vi "555集成定时器组成单稳态触发器.vi"() -> ()   [LabVIEW 2018]
panel:
  out "V":dbl
  out "毫秒计时值":u32
  out "波形图表":cluster{i16, i16}(graph)
  in  "确定按钮":bool
  in  "C值":dbl
  in  "R值":dbl
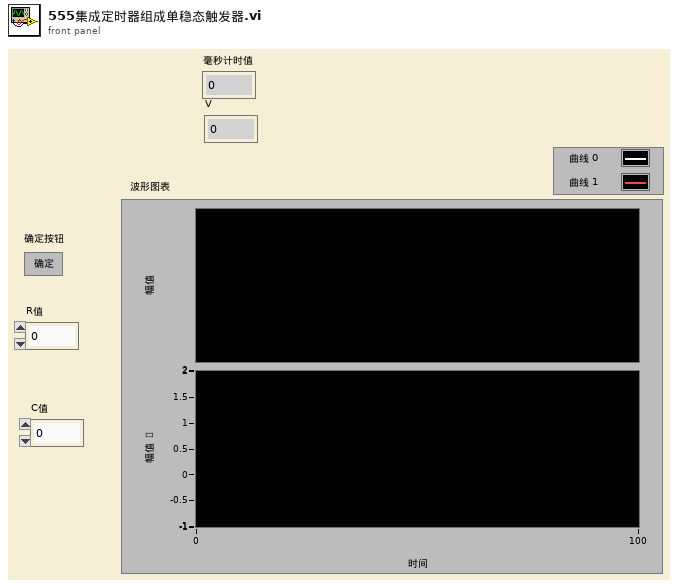
[diagram p1: front panel]
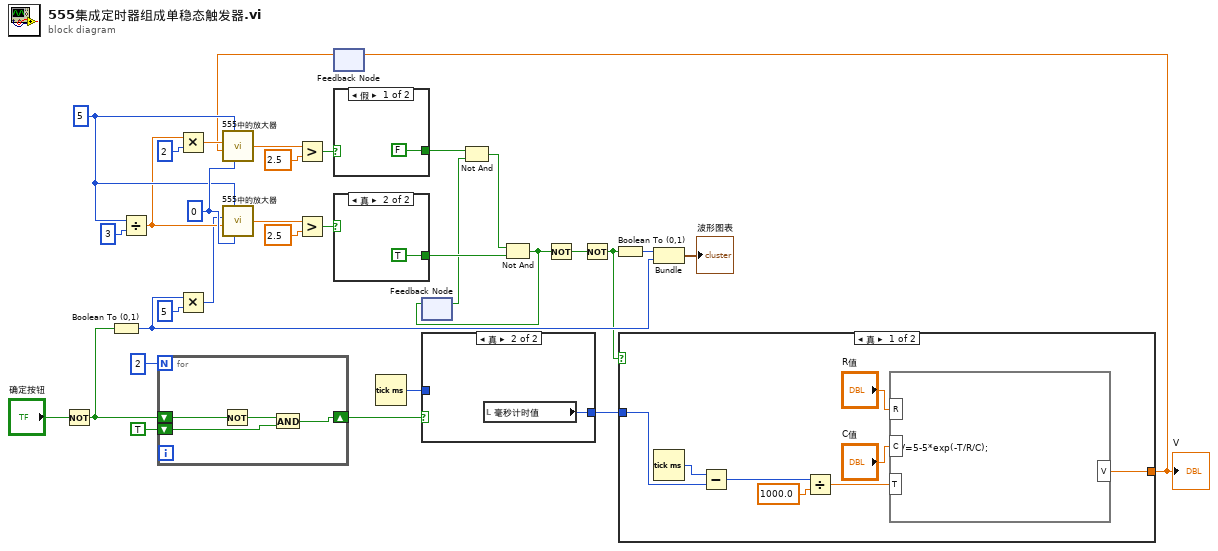
[diagram p0: block diagram]
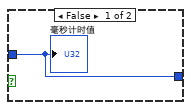
[diagram p2: hidden frame]
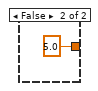
[diagram p3: hidden frame]
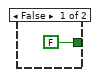
[diagram p4: hidden frame]
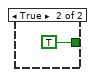
[diagram p5: hidden frame]
diagram:
  w21 = 0
  w20 = 5
  n1 = Not(x="确定按钮") -> (.not. x?=w1:bool)
  n2 = Boolean To (0,1)(Boolean=w1) -> (0, 1=w11:i16)
  n3 = Divide(x=w20, y=3) -> (x/y=w17:dbl)
  n4 = for {
    N: 2 -> [_]
    shift-right: [w34] -> w3
    shift-left: w1 -> [w37]
    shift-left: TRUE -> [w35]
    n5 = Not(x=w37) -> (.not. x?=w36:bool)
    n6 = And(x=w36, y=w35) -> (x .and. y?=w34:bool)
  }
  n7 = Multiply(x=w17, y=2) -> (x*y=w16:dbl)
  n8 = Multiply(x=w11, y=5) -> (x*y=w12:i32)
  n9 = call "555中的放大器.vi"("VCC"=w20, "IN+"=w12, "IN--"=w17, "--VCC"=w21) -> ("OUT"=w25:dbl)  [unwired: 4 in]
  n10 = Greater?(x=w25, y=2.5) -> (0:w30:bool)
  n11 = feedback #1() -> (w14:dbl)  [unwired: 1 in]
  n12 = call "555中的放大器.vi"("VCC"=w20, "IN+"=w16, "IN--"=w14, "--VCC"=w21) -> ("OUT"=w26:dbl)  [unwired: 4 in]
  n13 = Greater?(x=w26, y=2.5) -> (0:w32:bool)
  n14 = case shown="假" w32 {
    tunnel: [FALSE TRUE] -> w29
    frame False {
    }
    frame True {
    }
  }
  n15 = case shown="真" w30 {
    tunnel: [FALSE TRUE] -> w28
    frame False {
    }
    frame True {
    }
  }
  n16 = Tick Count (ms)() -> (millisecond timer value=w7:u32)
  n17 = feedback #2() -> (w24:bool)  [unwired: 1 in]
  n18 = case shown="真" w3 {
    tunnel: w7 -> [w42 _]
    tunnel: [w42 w43] -> w6
    frame False {
      "毫秒计时值" <- w42
    }
    frame True {
      n19 = local read "毫秒计时值"() -> (w43:u32)
    }
  }
  n20 = Not And(1:w24, 2:w29) -> (0:w27:bool)
  n21 = Not And(1:w28, 2:w27) -> (0:w22:bool)
  n22 = feedback-in #2(w22) -> ()
  n23 = Not(x=w22) -> (.not. x?=w23:bool)
  n24 = Not(x=w23) -> (.not. x?=w5:bool)
  n25 = Boolean To (0,1)(Boolean=w5) -> (0, 1=w10:i16)
  n26 = case shown="真" w5 {
    tunnel: w6 -> [w45 _]
    tunnel: [w44 5.0] -> w15
    frame True {
      n27 = Tick Count (ms)() -> (millisecond timer value=w47:u32)
      n28 = Subtract(x=w47, y=w45) -> (x-y=w48:u32)
      n29 = Divide(x=w48, y=1000.0) -> (x/y=w51:dbl)
      n30 = formula code="V=5-5*exp(-T/R/C);"("R"="R值", "C"="C值", "T"=w51) -> ("V"=w44:dbl)
    }
    frame False {
    }
  }
  "V" <- w15
  n31 = feedback-in #1(w15) -> ()
  n32 = Bundle(w10, w11) -> (→"波形图表":cluster{i16, i16})  [unwired: 1 in]
